vi "lock-in amplifier SR830 pump probe.vi"(7 "Integration time (ms)":dbl, 9 "Connection 2":refnum<visa-resource-name>, 11 "Connection":refnum<visa-resource-name>) -> (2 "pump probe signal":dbl)   [LabVIEW 2024]
uses:
  <vilib>/Analysis/baseanly.llb/Mean (DBL).vi
  <vilib>/Analysis/NI_AALBase.lvlib
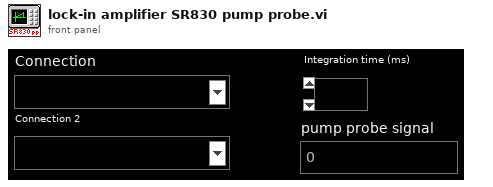
[diagram p1: front panel]
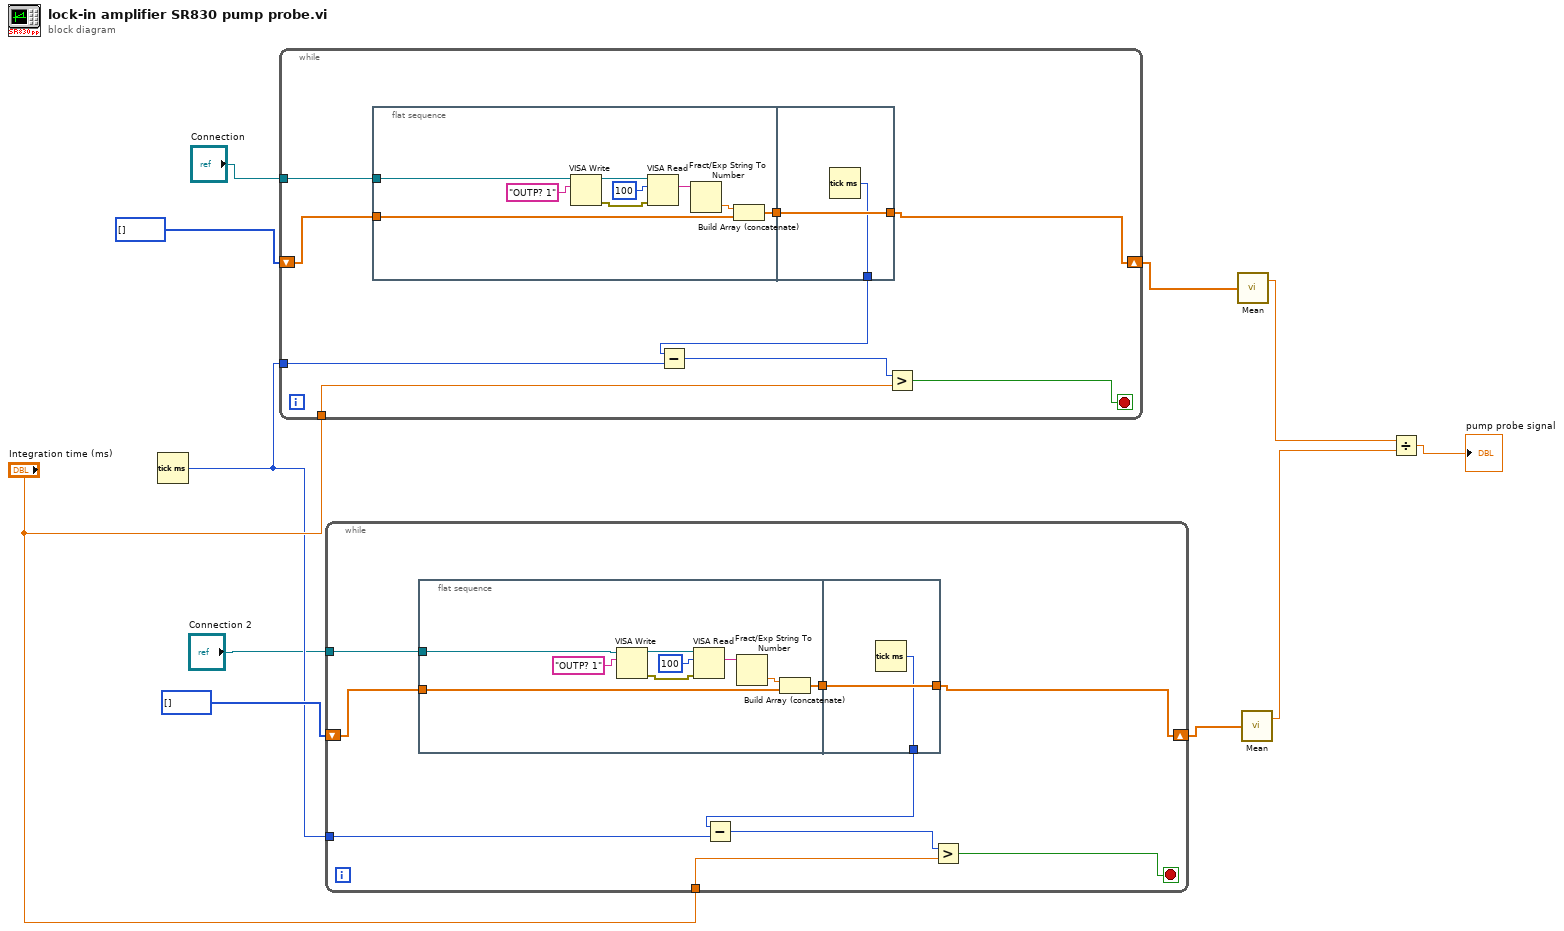
[diagram p0: block diagram]
diagram:
  n1 = Tick Count (ms)() -> (millisecond timer value=w8:u32)
  n2 = while {
    shift-right: [w20] -> w7
    shift-left: i32[] [] -> [w19]
    tunnel: w8 -> [w16]
    tunnel: "Integration time (ms)" -> [w13]
    tunnel: "Connection" -> [w12]
    stop <- w14 stop-if-true
    n3 = flat-sequence {
      tunnel: w19 -> [w23]
      tunnel: [w24] -> w18
      tunnel: w12 -> [w21]
      tunnel: [w31] -> w20
      tunnel: w18 -> [w31]
      tunnel: [w30] -> w17
      frame #0 {
        n4 = VISA Write(VISA resource name=w21, write buffer="OUTP? 1") -> (VISA resource name out=w29:refnum<visa-resource-name>, error out=w22:errorcluster)  [unwired: 1 in, 1 out]
        n5 = VISA Read(VISA resource name=w29, byte count=u32 100, error in (no error)=w22) -> (read buffer=w26:string)  [unwired: 3 out]
        n6 = Fract/Exp String To Number(string=w26) -> (number=w25:dbl)  [unwired: 3 in, 1 out]
        n7 = Build Array (concatenate)(w25, w23) -> (w24:dbl[])
      }
      frame #1 {
        n8 = Tick Count (ms)() -> (millisecond timer value=w30:u32)
      }
    }
    n9 = Subtract(x=w17, y=w16) -> (x-y=w15:u32)
    n10 = Greater?(x=w15, y=w13) -> (0:w14:bool)
  }
  n11 = while {
    shift-right: [w40] -> w6
    shift-left: i32[] [] -> [w39]
    tunnel: w8 -> [w36]
    tunnel: "Integration time (ms)" -> [w33]
    tunnel: "Connection 2" -> [w32]
    stop <- w34 stop-if-true
    n12 = flat-sequence {
      tunnel: w39 -> [w43]
      tunnel: [w44] -> w38
      tunnel: w32 -> [w41]
      tunnel: [w51] -> w40
      tunnel: w38 -> [w51]
      tunnel: [w50] -> w37
      frame #0 {
        n13 = VISA Write(VISA resource name=w41, write buffer="OUTP? 1") -> (VISA resource name out=w49:refnum<visa-resource-name>, error out=w42:errorcluster)  [unwired: 1 in, 1 out]
        n14 = VISA Read(VISA resource name=w49, byte count=u32 100, error in (no error)=w42) -> (read buffer=w46:string)  [unwired: 3 out]
        n15 = Fract/Exp String To Number(string=w46) -> (number=w45:dbl)  [unwired: 3 in, 1 out]
        n16 = Build Array (concatenate)(w45, w43) -> (w44:dbl[])
      }
      frame #1 {
        n17 = Tick Count (ms)() -> (millisecond timer value=w50:u32)
      }
    }
    n18 = Subtract(x=w37, y=w36) -> (x-y=w35:u32)
    n19 = Greater?(x=w35, y=w33) -> (0:w34:bool)
  }
  n20 = call-poly <vilib>:"Mean.vi"("X"=w7) -> ("mean"=w5:dbl)  [unwired: 1 out]
  n21 = call-poly <vilib>:"Mean.vi"("X"=w6) -> ("mean"=w4:dbl)  [unwired: 1 out]
  n22 = Divide(x=w5, y=w4) -> (x/y=→"pump probe signal":dbl)
